vi "setUp.vi"(8 "error in (no error)":errorcluster, 11 "reference in":refnum<class "Get Chamber Status.lvclass">) -> (0 "error out":errorcluster, 3 "reference out":refnum<class "Get Chamber Status.lvclass">)   [LabVIEW 2018, in "Get Chamber Status.lvclass"]
doc: "setUp runs prior to the test method during test execution. Use this method to initialize any object data required by your tests."
uses:
  Get Chamber Status.lvclass
  Libraries/Thermal Chamber Response Simulator/Thermal Chamber Response Simulator.lvlib
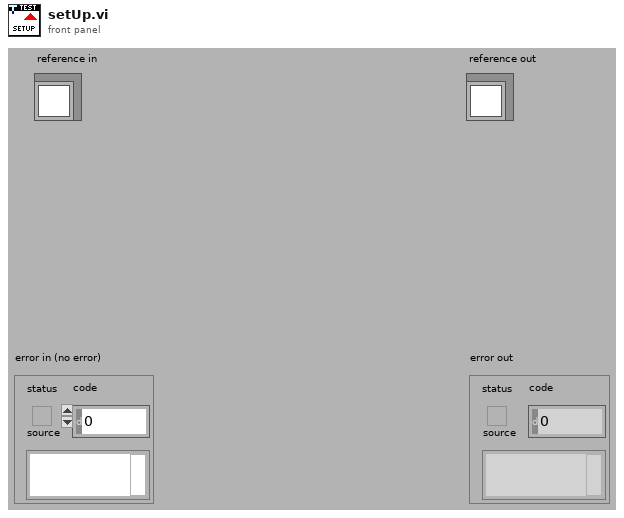
[diagram p1: front panel]
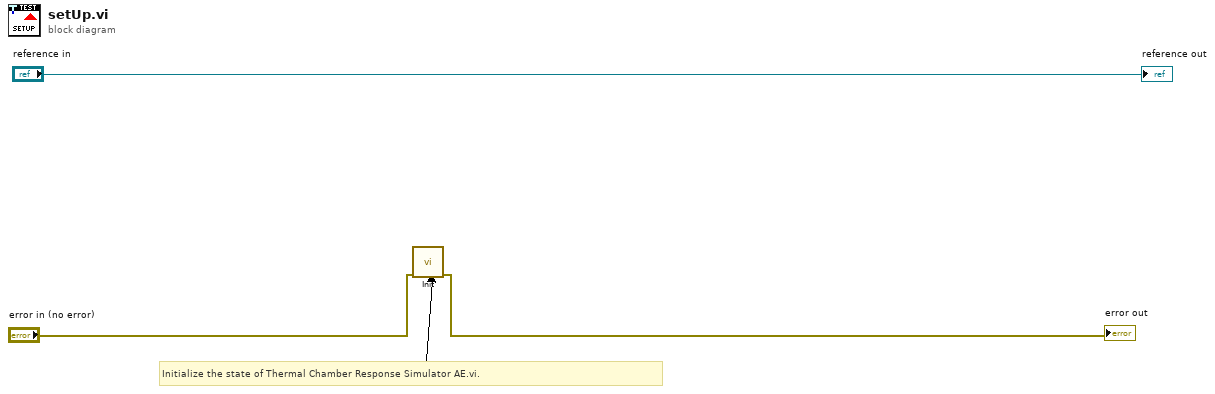
[diagram p0: block diagram]
diagram:
  # "Initialize the state of Thermal Chamber Response Simulator AE.vi."
  n1 = call "Init.vi"("error in (no error)"="error in (no error)") -> ("error out"=→"error out":errorcluster)  [unwired: 10 in]
  "reference out" <- "reference in"
